vi "查询产品生产时间.vi"(8 "error in (no error)":errorcluster, 10 "产品ID":string, 11 "ADODB._Connection In":refnum<k7>) -> (0 "error out":errorcluster, 1 "索引结果":bool, 2 "生产时间":string)   [LabVIEW 2013]
uses:
  <vilib>/Utility/error.llb/whitespace.ctl
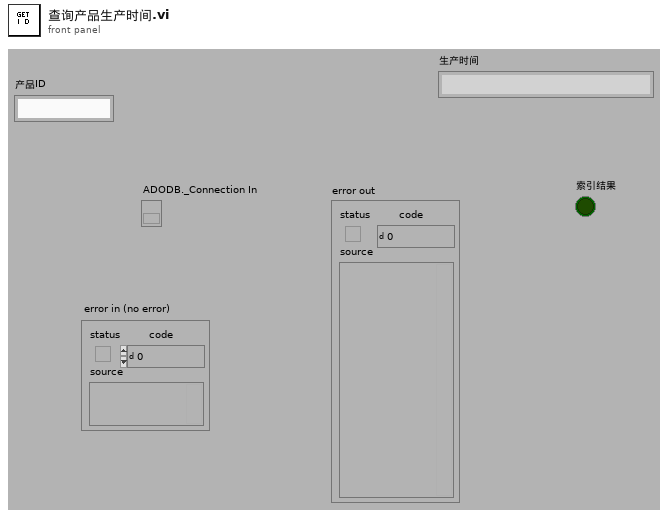
[diagram p1: front panel]
types:
  T1 = typedef "whitespace.ctl" = u16
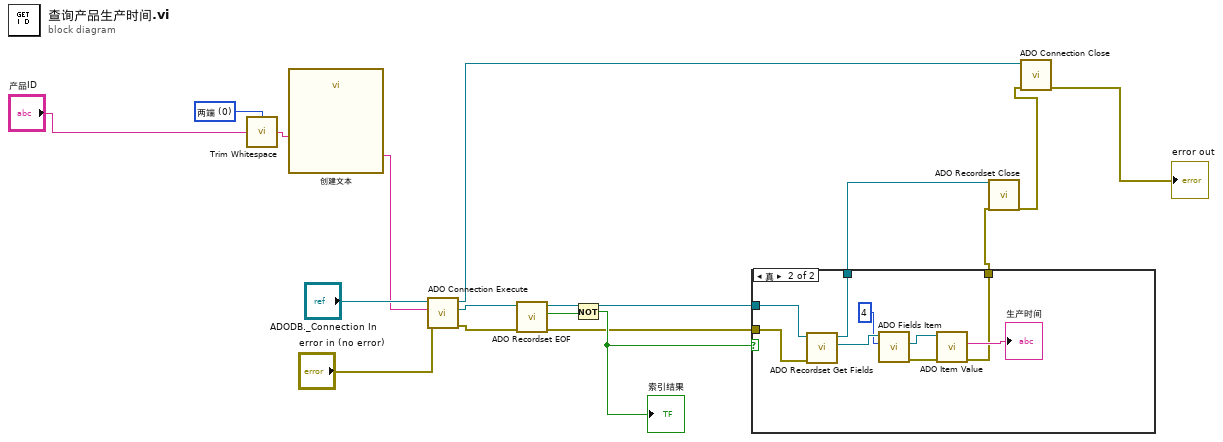
[diagram p0: block diagram]
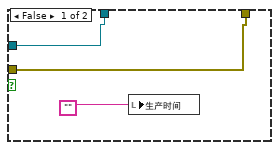
[diagram p2: hidden frame]
diagram:
  w12 = T1 0 items=["两端", "字符串首端", "字符串末端"] ("location (both)")
  n1 = call <vilib>:"Trim Whitespace.vi"("string"="产品ID", "location (both)"=w12) -> ("trimmed string"=w1:string)
  n2 = call "创建文本"("产品ID"=w1) -> ("Result"=w3:string)  [unwired: 13 in, 1 out]
  n3 = call "ADO Connection Execute.vi"("error in (no error)"="error in (no error)", "CommandText"=w3, "ADODB._Connection In"="ADODB._Connection In") -> ("error out"=w16:errorcluster, "RecordSet"=w17:refnum<k7>, "ADODB._Connection Out"=w13:refnum<k7>)  [unwired: 6 out]
  n4 = call "ADO Recordset EOF.vi"("error in (no error)"=w16, "ADODB._Recordset In"=w17) -> ("error out"=w8:errorcluster, "EOF"=w15:bool, "ADODB._Recordset Out"=w9:refnum<k7>)  [unwired: 7 out]
  n5 = Not(x=w15) -> (.not. x?=w10:bool)
  "索引结果" <- w10
  n6 = case shown="真" w10 {
    tunnel: w9 -> [w19 w29]
    tunnel: w8 -> [w20 w28]
    tunnel: [w19 w27] -> w7
    tunnel: [w20 w21] -> w6
    frame False {
      n7 = local write "生产时间"("") -> ()
    }
    frame True {
      n8 = call "ADO Recordset Get Fields.vi"("error in (no error)"=w28, "ADODB._Recordset In"=w29) -> ("Fields Out"=w26:refnum<k7>, "ADODB._Recordset Out"=w27:refnum<k7>)  [unwired: 8 out]
      n9 = call "ADO Fields Item.vi"("Index"=4, "Fields In"=w26) -> ("error out"=w24:errorcluster, "Item Out"=w23:refnum<k7>)  [unwired: 1 in, 7 out]
      n10 = call "ADO Item Value.vi"("error in (no error)"=w24, "Item In"=w23) -> ("error out"=w21:errorcluster, "Value"=→"生产时间":string)  [unwired: 8 out]
    }
  }
  n11 = call "ADO Recordset Close.vi"("ADODB._Recordset In"=w7, "error in (no error)"=w6) -> ("error out"=w14:errorcluster)  [unwired: 17 out]
  n12 = call "ADO Connection Close.vi"("error in (no error)"=w14, "ADODB._Connection In"=w13) -> ("error out"=→"error out":errorcluster)  [unwired: 9 out]
